vi "Delete All Attributes.vi"(8 "error in (no error)":errorcluster, 11 "Variant in":refnum<class "Variant.lvclass">) -> (0 "error out":errorcluster, 3 "Variant out":refnum<class "Variant.lvclass">)   [LabVIEW 2020, in "Data.lvlib" / "Variant.lvclass"]
doc: "Delete all attributes from the variant."
uses:
  Variant.lvclass
  Variant.lvclass/Variant.ctl
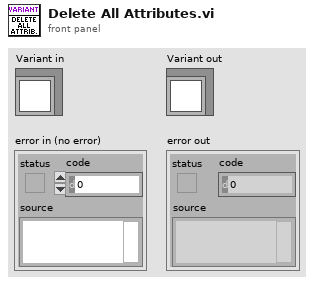
[diagram p1: front panel]
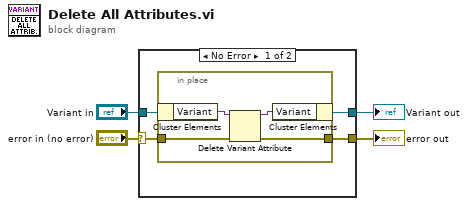
[diagram p0: block diagram]
diagram:
  n1 = case shown="No Error" "error in (no error)" {
    selector: "error in (no error)" -> [w6 w14]
    tunnel: [w5 w14] -> w2
    tunnel: [w7 w13] -> w1
    tunnel: "Variant in" -> [w8 w13]
    frame No Error {
      n2 = in-place {
        in-place-border: w6 -> [w11]
        in-place-border: [w10] -> w5
        n3 = in-place-cluster #1(w8) -> ("Variant"=w12:variant)
        n4 = Delete Variant Attribute(4:w11, 7:w12) -> (0:w10:errorcluster, 3:w9:variant)  [unwired: 1 in, 1 out]
        n5 = in-place-cluster #1("Variant"=w9) -> (w7:refnum<class "Variant.lvclass">)
      }
    }
    frame Error {
    }
  }
  "error out" <- w2
  "Variant out" <- w1
